vi "Find Item by Tag.vi"(8 "error in (no error)":errorcluster, 10 "Tag":string, 11 "Tree Manager in":refnum<class "Tree Manager.lvclass">) -> (0 "error out":errorcluster, 1 "Found?":bool, 2 "Data Item":refnum<class "Data Item.lvclass">, 3 "Tree Manager out":refnum<class "Tree Manager.lvclass">)   [LabVIEW 2018, in "VILab.lvlib" / "Tree Manager.lvclass"]
uses:
  Tree Manager.lvclass
  Data Item.lvclass
  Tree Manager.lvclass/Tree Manager.ctl
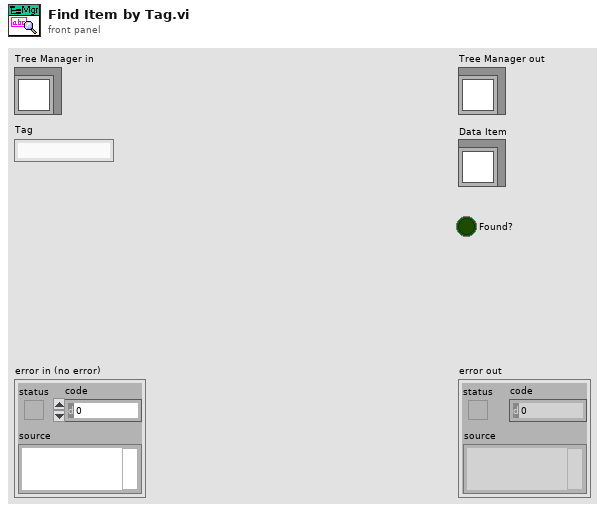
[diagram p1: front panel]
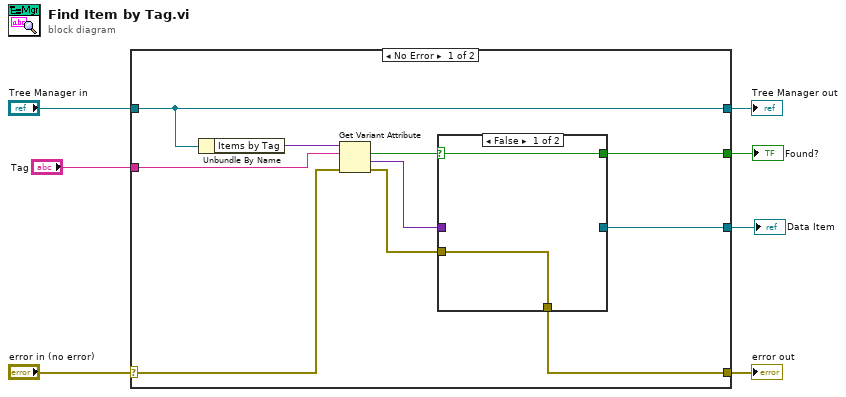
[diagram p0: block diagram]
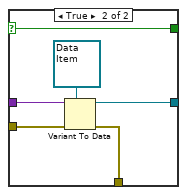
[diagram p2: hidden frame]
diagram:
  n1 = case shown="No Error" "error in (no error)" {
    selector: "error in (no error)" -> [w14 w27]
    tunnel: [w11 w27] -> w6
    tunnel: [w17 w26] -> w4
    tunnel: "Tree Manager in" -> [w17 w26]
    tunnel: "Tag" -> [w15 _]
    tunnel: [w9 _] -> w2
    tunnel: [w12 _] -> w1
    frame No Error {
      n2 = Unbundle By Name(w17) -> ("Items by Tag"=w16:variant)
      n3 = Get Variant Attribute(Variant=w16, name=w15, error in=w14) -> (found=w10:bool, value=w8:variant, error out=w13:errorcluster)  [unwired: 1 in, 1 out]
      n4 = case shown="False" w10 {
        selector: w10 -> [w19 w20]
        tunnel: w8 -> [_ w25]
        tunnel: w13 -> [w18 w23]
        tunnel: [_ w22] -> w12
        tunnel: [w18 w21] -> w11
        tunnel: [w19 w20] -> w9
        frame False {
        }
        frame True {
          n5 = Variant To Data(error in=w23, type=refnum<class "Data Item.lvclass"> refnum ("VILab.lvlib:Data Item.lvclass"), Variant=w25) -> (data=w22:refnum<class "Data Item.lvclass">, error out=w21:errorcluster)
        }
      }
    }
    frame Error {
    }
  }
  "error out" <- w6
  "Tree Manager out" <- w4
  "Found?" <- w2
  "Data Item" <- w1
